vi "LC1_OS_Main.vi"(0 "Network Settings 1":T2={"port (20000)"=18000, "Master IP"="48.26.87.212", "Master Address"=12345, "Outstation Address "=54321, " update rate"=50}, 1 "Analog Input":dbl[](array[numeric]), 5 "Settings Cluster":T1={"Default Variation:Analog Input Event (OBJ32)"=1, "Default Variation:Analog Input (OBJ30)"=1, "Default Variation:Binary Input (OBJ01)"=1, "Default Variation:Analog Output (OBJ40)"=4, "Default Variation:Binary Output Event (OBJ11)"=1, "Default Variation:Binary Output (OBJ10)"=1, "Default Variation:Analog Output Event (OBJ42)"=8, "Unsolicited Response Allowed"=FALSE, "Control:Select Timeout (ms)"=0, "Misc:Appl Confirmation Timeout"=0} {"Default Variation:Analog Output Event (OBJ42)" items=["32-bit without Time"=1, "16-bit without Time"=2, "32-bit with Time"=3, "16-bit with Time"=4, "Single-prec without Time"=5, "Double-prec without Time"=6, "Single-prec with Time"=7, "Double-prec with Time"=8]; "Default Variation:Binary Output (OBJ10)" items=["Packed Format"=1, "Output Status with Flags"=2]; "Default Variation:Binary Output Event (OBJ11)" items=["Status without Time"=1, "Status with Time"=2]; "Default Variation:Analog Output (OBJ40)" items=["32-bit with Flag"=1, "16-bit with Flag"=2, "Single-prec with Flag"=3, "Double-prec with Flag"=4]; "Default Variation:Binary Input (OBJ01)" items=["Packed Format"=1, "With Flags"=2]; "Default Variation:Analog Input (OBJ30)" items=["32-bit with Flag"=1, "16-bit with Flag"=2, "32-bit without Flag"=3, "16-bit without Flag"=4, "Single-prec with Flag"=5, "Double-prec with Flag"=6]; "Default Variation:Analog Input Event (OBJ32)" items=["32-bit without Time"=1, "16-bit without Time"=2, "32-bit with Time"=3, "16-bit with Time"=4, "Single-prec without Time"=5, "Double-prec without Time"=6, "Single-prec with Time"=7, "Double-prec with Time"=8]}, 7 "DNP3 DataMap 1":T3={"Binary Output Points"=1, "Binary Input Points"=0, "Analog Output Points"=7, "Analog Input Points"=6}, 9 "OS_Reset":bool, 11 "OS_Enable":bool, 12 "DNP3 Session Input":T4) -> (3 "Analog Output":dbl[](array[numeric]), 4 "OS_DNP3_Settings_Changed":bool, 8 "Connected?":bool, 14 "DNP3 Session":T4)   [LabVIEW 2016, in "DNP3_Outstation_Template.lvlib"]
doc: "-----------------------------------------------------------------------------------------------------------------------\nCopyright <2019> <The University of Tennessee at Knoxville and the University of Tennessee Research Foundation>\nThis software is released under BSD-3 a\nhttps://opensource.org/licenses/BSD-3-Clause \nAdditional license options available at https://utrf.tennessee.edu/industry/sample-agreements/\n-----------------------------------------------------------------------------------------------------------------------"
uses:
  DNP3_Outstation_Template.lvlib
  <vilib>/DNP3/DNP3_Common/crob.ctl
  <vilib>/DNP3/DNP3_Common/crob_ctrl.ctl
  <vilib>/DNP3/DNP3_Common/Create Channel (IP Networking).vi
  <vilib>/DNP3/DNP3_Outstation/Read Analog Output.vi
  <vilib>/DNP3/DNP3_Outstation/Write Analog Input.vi
  <vilib>/DNP3/DNP3_Outstation/Read Binary Output.vi
  <vilib>/DNP3/DNP3_Outstation/Write Binary Input.vi
  <vilib>/DNP3/DNP3_Common.lvlib
  <vilib>/DNP3/DNP3_Outstation.lvlib
  <resource>/objmgr/dnp3.rc
panel:
  out "OS_Reset_Succesful":bool
  out "OS_Reset_Ind":bool
  out "OS_DNP3_Settings_Initial":T1
  out "OS_Network_Settings_Initial":T2
  out "DNP3 DataMap_Initial":T3={"Binary Output Points"=1, "Binary Input Points"=0, "Analog Output Points"=7, "Analog Input Points"=6}
  out "Reset?":T5[](array[typedef]) {"Control" items=["Nul"=0, "Pulse On"=1, "Pulse Off"=2, "Latch On"=3, "Latch Off"=4, "Close"=65, "Trip"=129]}
  out "x > y?":bool
  out "Analog Input Points":u16 max=32
  out "Analog Output Points":u16 max=32
  out "Binary Input Points":u16 max=32
  out "Binary Output Points":u16 max=32
  out "Reset Cycles":i32
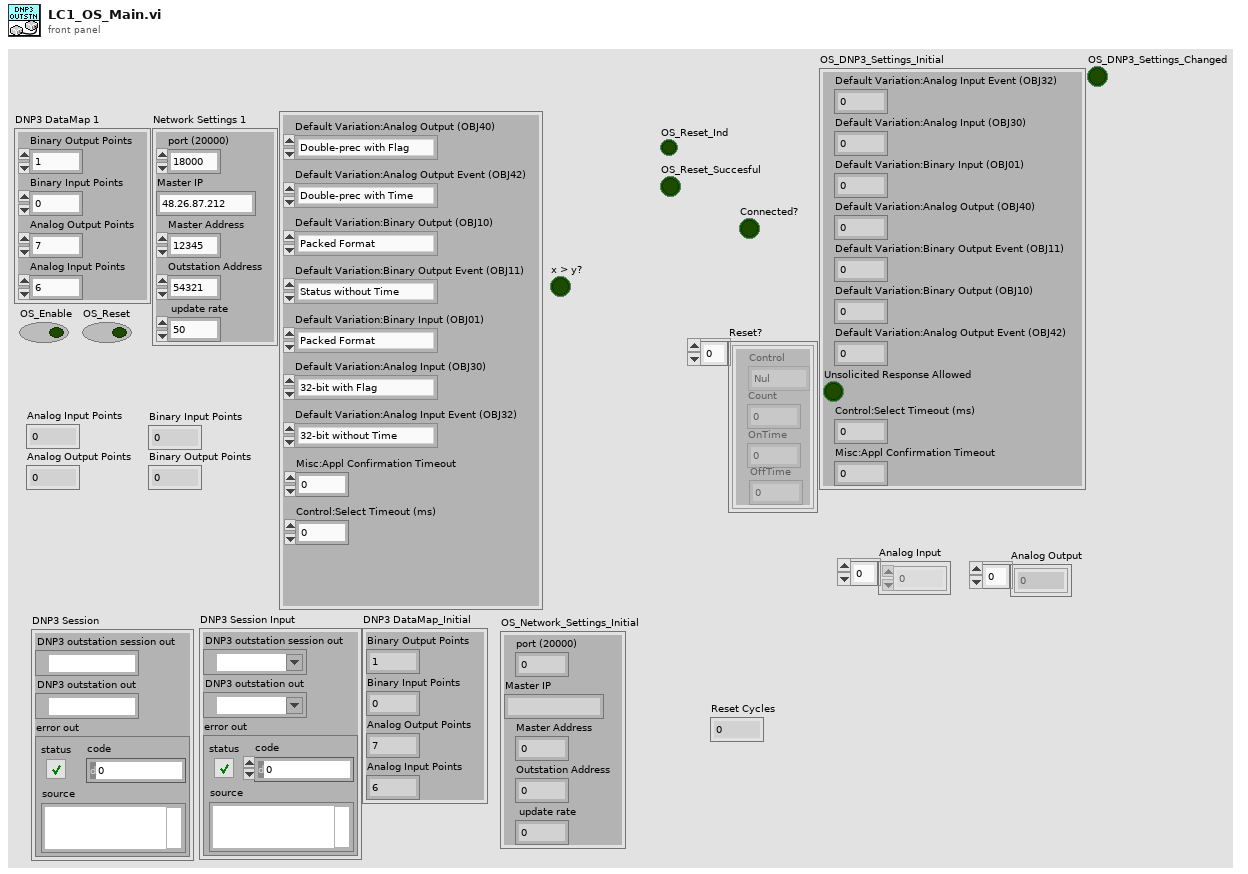
[diagram p1: front panel]
types:
  T1 = cluster{"Default Variation:Analog Input Event (OBJ32)":u8, "Default Variation:Analog Input (OBJ30)":u8, "Default Variation:Binary Input (OBJ01)":u8, "Default Variation:Analog Output (OBJ40)":u8, "Default Variation:Binary Output Event (OBJ11)":u8, "Default Variation:Binary Output (OBJ10)":u8, "Default Variation:Analog Output Event (OBJ42)":u8, "Unsolicited Response Allowed":bool, "Control:Select Timeout (ms)":u32, "Misc:Appl Confirmation Timeout":u32}
  T2 = cluster{"port (20000)":u16, "Master IP":string, "Master Address":u16, "Outstation Address ":u16, " update rate":u32}
  T3 = cluster{"Binary Output Points":u16, "Binary Input Points":u16, "Analog Output Points":u16, "Analog Input Points":u16}
  T4 = cluster{"DNP3 outstation session out":refnum<k21>, "DNP3 outstation out":refnum<k21>, "error out":errorcluster}
  T5 = typedef "DNP3_Common.lvlib/crob.ctl" = cluster{"OnTime":u32, "Count":u8, "OffTime":u32, "Control":T6}
  T6 = typedef "DNP3_Common.lvlib/crob_ctrl.ctl" = u8
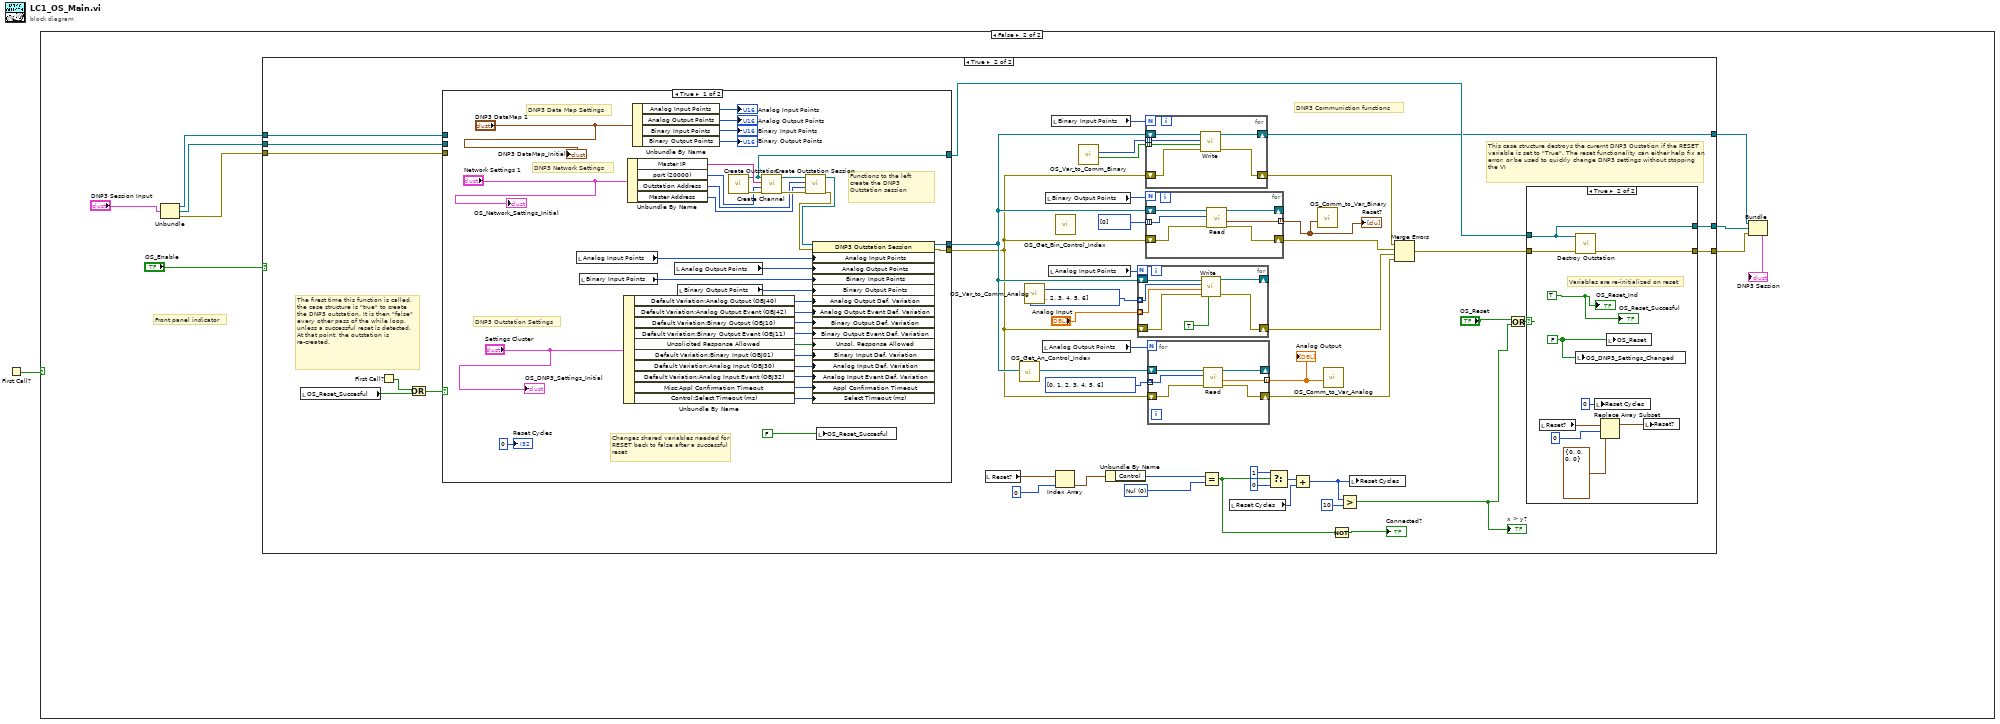
[diagram p0: block diagram]
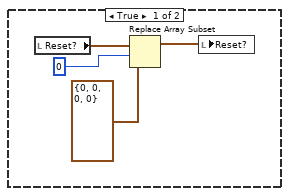
[diagram p2: hidden frame]
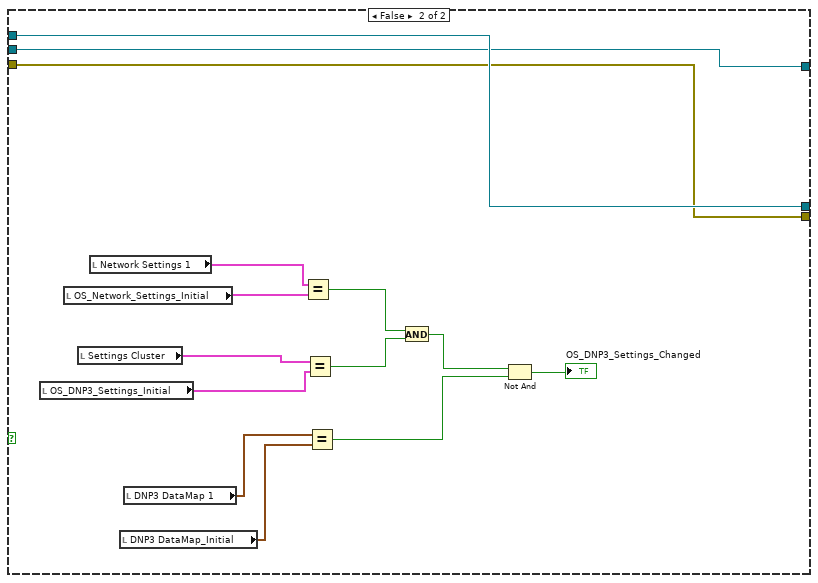
[diagram p5: hidden frame]
diagram:
  n1 = First Call?() -> (First Call?: T/F=w1:bool)
  n2 = case shown="False" w1 {
    frame True {
      n3 = local read "Reset?"() -> (w3:T5[])
      n4 = Replace Array Subset(array=w3, new element=T5 {"OnTime"=0, "Count"=0, "OffTime"=0, "Control"=0} ("new element/subarray"), index=0) -> (w2:T5[])
      n5 = local write "Reset?"(w2) -> ()
    }
    frame False {
      # "Front panel indicator"
      n6 = Unbundle("DNP3 Session Input") -> ("DNP3 outstation session out"=w8:refnum<k21>, "DNP3 outstation out"=w7:refnum<k21>, "error out"=w6:errorcluster)
      n7 = case shown="True" "OS_Enable" {
        tunnel: w8 -> [w17 w56]
        tunnel: w7 -> [w16 w55]
        tunnel: [w17 w54] -> w13
        tunnel: [w16 w53] -> w12
        tunnel: [w15 w52] -> w11
        tunnel: w6 -> [w15 w51]
        frame False {
        }
        frame True {
          w46 = T6 0 items=["Nul"=0, "Pulse On"=1, "Pulse Off"=2, "Latch On"=3, "Latch Off"=4, "Close"=65, "Trip"=129] ("y")
          # "DNP3 Communiction functions"
          # "This case structure destroys the curernt DNP3 Oustation if the RESET variable is set to \"True\". The reset functionality can either help fix an error, or be used to quickly change DNP3 settings without stopping the VI"
          # "The firest time this function is called, the case structure is \"true\" to create the DNP3 outstation. It is then \"false\" every other pass of the while loop, unless a successful reset is detected. At that point, the outstation is re-created."
          n8 = local read "OS_Reset_Succesful"() -> (w23:bool)
          n9 = First Call?() -> (First Call?: T/F=w57:bool)
          n10 = Or(x=w57, y=w23) -> (x .or. y?=w58:bool)
          n11 = case shown="True" w58 {
            tunnel: [w107 w148] -> w62
            tunnel: [w106 w146] -> w61
            tunnel: [w105 w147] -> w60
            tunnel: w56 -> [_ w148]
            tunnel: w55 -> [_ w147]
            tunnel: w51 -> [_ w146]
            frame True {
              # "Functions to the left create the DNP3 Outstation session"
              # "DNP3 Data Map Settings"
              # "DNP3 Network Settings"
              # "DNP3 Outstation Settings"
              # "Changes shared variables needed for RESET back to false after a successful reset"
              n12 = local read "Analog Input Points"() -> (w110:u16)
              n13 = local read "Binary Input Points"() -> (w112:u16)
              n14 = Unbundle By Name("Settings Cluster") -> ("Default Variation:Analog Output (OBJ40)"=w114:u8, "Default Variation:Analog Output Event (OBJ42)"=w115:u8, "Default Variation:Binary Output (OBJ10)"=w116:u8, "Default Variation:Binary Output Event (OBJ11)"=w117:u8, "Unsolicited Response Allowed"=w118:bool, "Default Variation:Binary Input (OBJ01)"=w119:u8, "Default Variation:Analog Input (OBJ30)"=w120:u8, "Default Variation:Analog Input Event (OBJ32)"=w121:u8, "Misc:Appl Confirmation Timeout"=w122:u32, "Control:Select Timeout (ms)"=w123:u32)
              n15 = Unbundle By Name("Network Settings 1") -> ("Master IP"=w131:string, "port (20000)"=w130:u16, "Outstation Address"=w129:u16, "Master Address"=w128:u16)
              n16 = Unbundle By Name("DNP3 DataMap 1") -> ("Analog Input Points"=→"Analog Input Points":u16, "Analog Output Points"=→"Analog Output Points":u16, "Binary Input Points"=→"Binary Input Points":u16, "Binary Output Points"=→"Binary Output Points":u16)
              n17 = local read "Analog Output Points"() -> (w111:u16)
              n18 = local read "Binary Output Points"() -> (w113:u16)
              n19 = call <vilib>:"Create Outstation.vi"() -> ("error out"=w134:errorcluster, "DNP3 outstation out"=w105:refnum<k21>)  [unwired: 10 in]
              n20 = call-poly <vilib>:"Create Channel.vi"("error in (no error)"=w134, "port (20000)"=w130, "IP"=w131, "DNP3 outstation"=w105) -> ("error out"=w133:errorcluster, "DNP3 channel out"=w132:refnum<k21>)  [unwired: 6 in]
              n21 = call <vilib>:"Create Outstation Session.vi"("error in (no error)"=w133, "destination"=w128, "source"=w129, "DNP3 channel"=w132) -> ("error out"=w109:errorcluster, "DNP3 outstation session out"=w108:refnum<k21>)  [unwired: 6 in]
              n22 = property class="DNP3 Outstation Session"(reference=w108, error in=w109, "Analog Input Points"=w110, "Analog Output Points"=w111, "Binary Input Points"=w112, "Binary Output Points"=w113, "Analog Output Def. Variation"=w114, "Analog Output Event Def. Variation"=w115, "Binary Output Def. Variation"=w116, "Binary Output Event Def. Variation"=w117, "Unsol. Response Allowed"=w118, "Binary Input Def. Variation"=w119, "Analog Input Def. Variation"=w120, "Analog Input Event Def. Variation"=w121, "Appl Confirmation Timeout"=w122, "Select Timeout (ms)"=w123) -> (reference out=w107:refnum<k21>, error out=w106:errorcluster)
              n23 = local write "OS_Reset_Succesful"(FALSE ("Reset Outstation")) -> ()
              "Reset Cycles" <- 0 ("Reset Cycles")
              "DNP3 DataMap_Initial" <- "DNP3 DataMap 1"
              "OS_Network_Settings_Initial" <- "Network Settings 1"
              "OS_DNP3_Settings_Initial" <- "Settings Cluster"
            }
            frame False {
              n24 = local read "OS_DNP3_Settings_Initial"() -> (w137:T1)
              n25 = local read "OS_Network_Settings_Initial"() -> (w136:T2)
              n26 = local read "Settings Cluster"() -> (w138:T1)
              n27 = local read "Network Settings 1"() -> (w135:T2)
              n28 = local read "DNP3 DataMap_Initial"() -> (w139:T3)
              n29 = local read "DNP3 DataMap 1"() -> (w140:T3)
              n30 = Equal?(x=w135, y=w136) -> (x = y?=w144:bool)
              n31 = Equal?(x=w138, y=w137) -> (x = y?=w143:bool)
              n32 = Equal?(x=w140, y=w139) -> (x = y?=w145:bool)
              n33 = And(x=w144, y=w143) -> (x .and. y?=w142:bool)
              n34 = Not And(1:w145, 2:w142) -> (0:→"OS_DNP3_Settings_Changed":bool)
            }
          }
          n35 = local read "Reset?"() -> (w41:T5[])
          n36 = call "OS_Get_An_Control_Index.vi"() -> ()  [unwired: 11 in, 1 out]
          n37 = call "OS_Var_to_Comm_Analog.vi"() -> ()  [unwired: 10 in, 2 out]
          n38 = local read "Analog Output Points"() -> (w32:u16)
          n39 = local read "Binary Output Points"() -> (w34:u16)
          n40 = local read "Analog Input Points"() -> (w33:u16)
          n41 = local read "Binary Input Points"() -> (w35:u16)
          n42 = Index Array(array=w41, index=0) -> (element=w39:T5)
          n43 = call "OS_Get_Bin_Control_Index.vi"() -> ()  [unwired: 11 in, 1 out]
          n44 = call "OS_Var_to_Comm_Binary.vi"() -> ("Array 3"=w27:bool[], "Array"=w25:u16[])  [unwired: 10 in]
          n45 = Unbundle By Name(w39) -> ("Control"=w38:T6)
          n46 = for {
            N: w33 -> [_]
            shift-right: [w78] -> w29
            shift-left: w61 -> [w79]
            shift-right: [w80] -> _
            shift-left: w62 -> [w81]
            tunnel: "Analog Input" -> [w76] mode=indexing
            tunnel: u16[] [0, 1, 2, 3, 4, 5, 6] ("Array") -> [w75] mode=indexing
            n47 = call-poly <vilib>:"Write.vi"("generate event? (false)"=TRUE, "error in (no error)"=w79, "value"=w76, "point index"=w75, "DNP3 outstation session"=w81) -> ("error out"=w78:errorcluster, "DNP3 outstation session"=w80:refnum<k21>)  [unwired: 5 in]
          }
          n48 = for {
            N: w35 -> [_]
            tunnel: w27 -> [w87] mode=indexing
            shift-right: [w85] -> w54
            shift-left: w62 -> [w86]
            shift-right: [w83] -> w31
            shift-left: w61 -> [w84]
            tunnel: w25 -> [w82] mode=indexing
            n49 = call-poly <vilib>:"Write.vi"("error in (no error)"=w84, "value"=w87, "point index"=w82, "DNP3 outstation session"=w86) -> ("error out"=w83:errorcluster, "DNP3 outstation session"=w85:refnum<k21>)  [unwired: 6 in]
          }
          n50 = for {
            N: w34 -> [_]
            shift-right: [w74] -> _
            shift-left: w62 -> [w73]
            shift-right: [w71] -> w30
            shift-left: w61 -> [w72]
            tunnel: [w70] -> w26 mode=indexing
            tunnel: u16[] [0] ("Array") -> [w69] mode=indexing
            n51 = call-poly <vilib>:"Read.vi"("error in (no error)"=w72, "point index"=w69, "DNP3 outstation session"=w73) -> ("error out"=w71:errorcluster, "CROB value"=w70:T5, "DNP3 outstation session"=w74:refnum<k21>)  [unwired: 4 in, 2 out]
          }
          "Reset?" <- w26
          n52 = for {
            N: w32 -> [_]
            shift-right: [w66] -> _
            shift-left: w62 -> [w67]
            shift-right: [w64] -> w28
            shift-left: w61 -> [w65]
            tunnel: [w68] -> w24 mode=indexing
            tunnel: u16[] [0, 1, 2, 3, 4, 5, 6] ("Array") -> [w63] mode=indexing
            n53 = call-poly <vilib>:"Read.vi"("error in (no error)"=w65, "point index"=w63, "DNP3 outstation session"=w67) -> ("error out"=w64:errorcluster, "current value"=w68:dbl, "DNP3 outstation session"=w66:refnum<k21>)  [unwired: 4 in, 2 out]
          }
          "Analog Output" <- w24
          n54 = Equal?(x=w38, y=w46) -> (x = y?=w42:bool)
          n55 = local read "Reset Cycles"() -> (w45:i32)
          n56 = Select(t=1, s=w42, f=0) -> (s? t:f=w47:i32)
          n57 = Add(x=w47, y=w45) -> (x+y=w43:i32)
          n58 = call "OS_Comm_to_Var_Binary.vi"("Array 3"=w26) -> ()  [unwired: 11 in]
          n59 = call "OS_Comm_to_Var_Analog.vi"("Array"=w24) -> ()  [unwired: 11 in]
          n60 = Not(x=w42) -> (.not. x?=→"Connected?":bool)
          n61 = Greater?(x=w43, y=10) -> (0:w37:bool)
          "x > y?" <- w37
          n62 = local write "Reset Cycles"(w43) -> ()
          n63 = Merge Errors(w31, w30, w29, w28) -> (w59:errorcluster)
          n64 = Or(x="OS_Reset", y=w37) -> (x .or. y?=w50:bool)
          n65 = case shown="True" w50 {
            tunnel: w60 -> [w88 w97]
            tunnel: w59 -> [w89 w99]
            tunnel: [w89 w98] -> w52
            tunnel: [w88 w97] -> w53
            frame False {
            }
            frame True {
              w90 = FALSE ("Comm_Reset")
              w91 = TRUE ("OS1 TX/RX 2")
              # "Variables are re-initialized on reset"
              n66 = local read "Reset?"() -> (w94:T5[])
              n67 = local write "OS_DNP3_Settings_Changed"(w90) -> ()
              n68 = call <vilib>:"Destroy Outstation.vi"("error in (no error)"=w99, "DNP3 outstation"=w97) -> ("error out"=w98:errorcluster)  [unwired: 9 in]
              n69 = local write "Reset Cycles"(0 ("Reset Cycles")) -> ()
              n70 = Replace Array Subset(array=w94, new element=T5 {"OnTime"=0, "Count"=0, "OffTime"=0, "Control"=0} ("new element/subarray"), index=0) -> (w95:T5[])
              n71 = local write "OS_Reset"(w90) -> ()
              n72 = local write "Reset?"(w95) -> ()
              "OS_Reset_Ind" <- w91
              "OS_Reset_Succesful" <- w91
            }
          }
        }
      }
      n73 = Bundle("DNP3 outstation session out"=w13, "DNP3 outstation out"=w12, "error out"=w11) -> (→"DNP3 Session":T4)  [unwired: 1 in]
    }
  }
